vi "Teleop.vi"(10 "Match Info":T1={"Autonomous Elapsed Seconds"=0.0, "TeleOp Elapsed Seconds"=0.0, "Disabled Elapsed Seconds"=0.0, "Visited Autonomous"=FALSE, "Visited TeleOp"=FALSE, "Visited Disabled"=FALSE, "Autonomous Settings"={"Autonomous Style"=enum."Independent", "VI Refnum"=refnum}}, 11 "Call Context":T2) -> ()   [LabVIEW 2014]
doc: "This VI is called for each TeleOp packet received from the DS where the robot is not disabled. It is often used to read from the joysticks and update I/O or to update setpoints for timed control loops. It should complete and return within 20 milliseconds or it may miss DS packets."
uses:
  <vilib>/Rock Robotics/WPI/DriverStation/WPI_DriverStationDerivedRobotMode.ctl
  <vilib>/Rock Robotics/WPI/DriverStation/WPI_DriverStationMatch Info.ctl
  Robot Global Data.vi
  <vilib>/Rock Robotics/WPI/RobotDrive/WPI_RobotDriveMecanumDrive_Cartesian.vi
  <vilib>/Rock Robotics/WPI/Solenoid/Deprecated/WPI_SolenoidSetBool.vi
  <vilib>/Rock Robotics/Network Tables/SD Write Numeric Array.vi
  <vilib>/addons/control/pid/NI_PID_pid.lvlib
  <vilib>/addons/control/pid/pid.llb/PID (DBL).vi
  PID Target Angle.vi
  <vilib>/Rock Robotics/Network Tables/SD Read Boolean.vi
  <vilib>/Rock Robotics/Network Tables/SD Read Number.vi
  <vilib>/Rock Robotics/Network Tables/SD Write Number.vi
panel:
  out "PID Raw Angle":dbl
  out "PID Target":dbl
  out "Joystick Z'":dbl
  out "Joystick Y'":dbl
  out "Joystick X'":dbl
  in  "Lift Encoder Target":dbl
  out "In-Range":bool
  out "Lift Stopped":bool
  out "Lift Direction":bool
  out "Lift Encoder Distance":dbl
  out "Lift Encoder Rate":dbl
  out "Bottom Limit":bool
  out "Top Limit":bool
  out "Wheel Stopped":bool
  out "Wheel Direction":bool
  out "Wheel Encoder Distance":dbl
  out "Wheel Encoder Rate":dbl
  out "Lift Motor Speed":dbl
  out "Angle":dbl(knob) scale=0.0..360.0
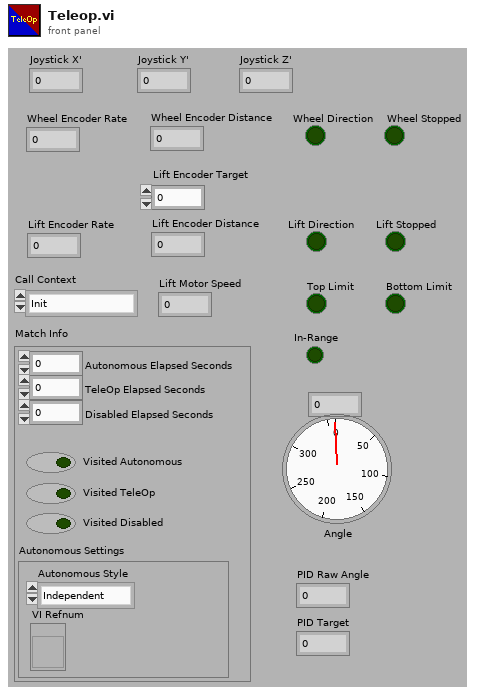
[diagram p1: front panel]
types:
  T1 = typedef "WPI_DriverStationMatch Info.ctl" = cluster{"Autonomous Elapsed Seconds":dbl, "TeleOp Elapsed Seconds":dbl, "Disabled Elapsed Seconds":dbl, "Visited Autonomous":bool, "Visited TeleOp":bool, "Visited Disabled":bool, "Autonomous Settings":cluster{"Autonomous Style":enum16{"Iterative", "Independent"}, "VI Refnum":refnum<vi>}}
  T2 = typedef "WPI_DriverStationDerivedRobotMode.ctl" = enum16{"Init", "Execute", "Stop"}
  T3 = typedef "WPI_GyroDevRef.ctl" = cluster{"DevStatus":errorcluster, "Analog Module":T4, "Analog Channel":T5, "Offset":dbl, "Gain (VoltsPerDegree/Second)":dbl}
  T4 = typedef "FPGA_TypedefAnalogModule.ctl" = enum16{"Controller 1"}
  T5 = typedef "FPGA_AIChannel.ctl" = enum8{"AI 0", "AI 1", "AI 2", "AI 3", "AI MXP 0", "AI MXP 1", "AI MXP 2", "AI MXP 3", "Invalid"}
  T6 = typedef "WPI_JoystickDevRef.ctl" = cluster{"Device":T7}
  T7 = typedef "WPI_JoystickDeviceEnum.ctl" = enum16{"USB 0", "USB 1", "USB 2", "USB 3", "USB 4", "USB 5"}
  T8 = typedef "WPI_SolenoidDevRef.ctl" = cluster{"DevStatus":errorcluster, "Pneumatics Control Module":u8, "Forward Solenoid Channel":T9, "Reverse Solenoid Channel":T9}
  T9 = typedef "WPI_SolenoidChannel.ctl" = enum8{"Solenoid 0", "Solenoid 1", "Solenoid 2", "Solenoid 3", "Solenoid 4", "Solenoid 5", "Solenoid 6", "Solenoid 7", "Invalid"}
  T10 = cluster{"Buttons[0]":bool, "Buttons[1]":bool, "Buttons[2]":bool, "Buttons[3]":bool, "Buttons[4]":bool, "Buttons[5]":bool, "Buttons[6]":bool, "Buttons[7]":bool, "Buttons[8]":bool}
  T11 = typedef "WPI_EncoderDevRef.ctl" = cluster{"DevStatus":errorcluster, "EncoderIndex":T12, "CounterIndex":T13, "DistancePerCount":dbl, "Decoding Type":T14}
  T12 = typedef "FPGA_EncoderIdx.ctl" = enum8{"Enc 0", "Enc 1", "Enc 2", "Enc 3", "Enc 4", "Enc 5", "Enc 6", "Enc 7", "Invalid"}
  T13 = typedef "FPGA_CounterCtrSystemIndex.ctl" = enum8{"Ctr 0", "Ctr 1", "Ctr 2", "Ctr 3", "Ctr 4", "Ctr 5", "Ctr 6", "Ctr 7", "Invalid"}
  T14 = typedef "WPI_EncoderType.ctl" = enum16{"1x", "2x", "4x"}
  T15 = cluster{"proportional gain (Kc)":dbl, "integral time (Ti, min)":dbl, "derivative time (Td, min)":dbl}
  T16 = typedef "WPI_RobotDriveDevRef.ctl" = cluster{"DevStatus":errorcluster, "Motors[]":T17[], "Square Inputs":bool, "Max Output":dbl}
  T17 = typedef "WPI_MotorControlDeviceRef.ctl" = cluster{"DeviceStatus":errorcluster, "Type":T18, "PWM":cluster{"Controller":T19, "PWM Channel":T20, "DeadBand":T21}, "CAN":cluster{"Device Number":u8, "Control Mode":T22, "Semaphore":T23, "Max Vout":dbl, "TalonSRX Control Mode":T24}, "Invert":bool, "TransformRef":T25, "InvTransformRef":T25}
  T18 = typedef "WPI_MotorControlType.ctl" = enum16{"PWM", "CAN", "CANTalonSRX"}
  T19 = typedef "FPGA_TypedefDigitalModule.ctl" = enum16{"Controller 1"}
  T20 = typedef "FPGA_DIOPWMChannel.ctl" = enum8{"PWM 0", "PWM 1", "PWM 2", "PWM 3", "PWM 4", "PWM 5", "PWM 6", "PWM 7", "PWM 8", "PWM 9", "PWM MXP 0", "PWM MXP 1", "PWM MXP 2", "PWM MXP 3", "PWM MXP 4", "PWM MXP 5", "PWM MXP 6", "PWM MXP 7", "PWM MXP 8", "PWM MXP 9", "Invalid"}
  T21 = typedef "WPI_PWMDeadband.ctl" = cluster{"Name":string, "maxPositivePwm":i32, "minPositivePwm":i32, "centerPwm":i32, "maxNegativePwm":i32, "minNegativePwm":i32, "angularRange":u16}
  T22 = typedef "WPI_CANJaguar_ControlMode.ctl" = enum8{"Percent VBus", "Current", "Speed", "Position", "Voltage"}
  T23 = typedef "Semaphore RefNum" = refnum<k1>
  T24 = typedef "WPI_CANTalonSRX_APIControlMode.ctl" = enum8{"Percent VBus", "Speed", "Position", "Slave", "Unchanged / Invalid"}
  T25 = typedef "WPI_PWMTransform_ConPane.ctl" = refnum<vi>
  T26 = typedef "WPI_SwitchDevRef.ctl" = cluster{"DevStatus":errorcluster, "DIO Channel":T27, "Controller":T19, "CntIndex":T13, "Normally Closed":bool}
  T27 = typedef "FPGA_DIOChannel.ctl" = enum8{"DIO 0", "DIO 1", "DIO 2", "DIO 3", "DIO 4", "DIO 5", "DIO 6", "DIO 7", "DIO 8", "DIO 9", "DIO MXP 0", "DIO MXP 1", "DIO MXP 2", "DIO MXP 3", "DIO MXP 4", "DIO MXP 5", "DIO MXP 6", "DIO MXP 7", "DIO MXP 8", "DIO MXP 9", "DIO MXP 10", "DIO MXP 11", "DIO MXP 12", "DIO MXP 13", "DIO MXP 14", "DIO MXP 15", "Invalid"}
  T28 = cluster{"X":dbl, "Y":dbl, "Angle":dbl, "Magnitude":dbl}
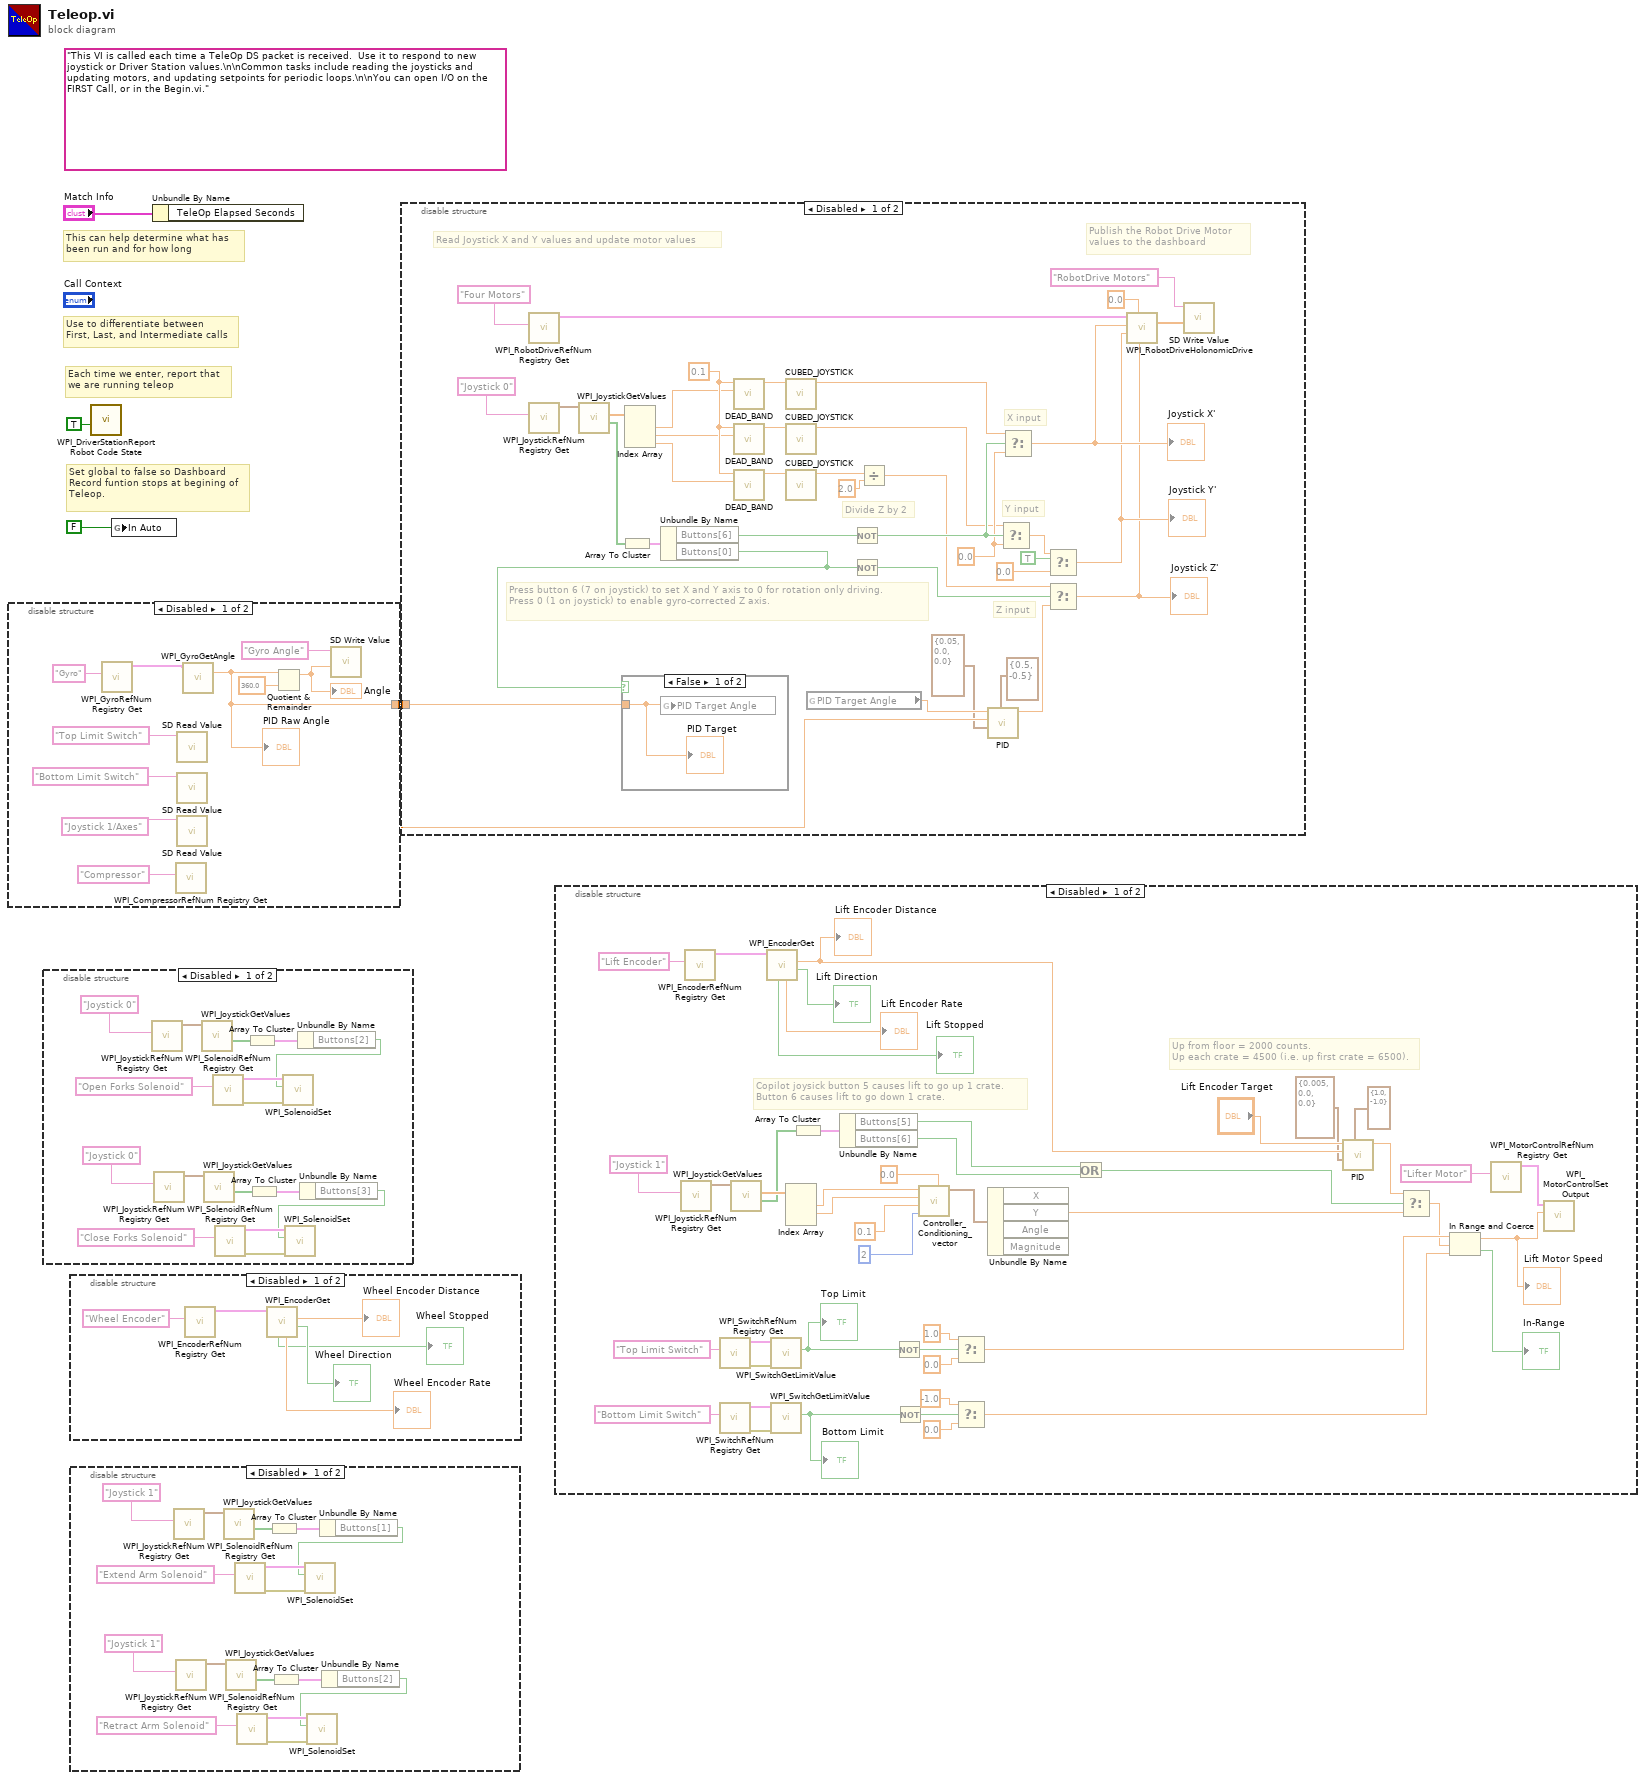
[diagram p0: block diagram]
diagram:
  (unwired) "This VI is called each time a TeleOp DS packet is received.  Use it to respond to new joystick or Driver Station values.\n\nCommon tasks include reading the joysticks and updating motors, and updating setpoints for periodic loops.\n\nYou can open I/O on the FIRST Call, or in the Begin.vi."
  # "Set global to false so Dashboard Record funtion stops at begining of Teleop."
  # "Each time we enter, report that\nwe are running teleop"
  # "Use to differentiate between\nFirst, Last, and Intermediate calls"
  # "This can help determine what has\nbeen run and for how long"
  n1 = disable-structure shown="Disabled" {
    disable-tunnel: [w6 _] -> w2
    frame Disabled {
      n2 = call <vilib>:"WPI_GyroRefNum Registry Get.vi"("refnum name"="Gyro") -> ("GyroDevRef"=w8:T3)  [unwired: 9 in, 1 out]
      n3 = call <vilib>:"WPI_CompressorRefNum Registry Get.vi"("refnum name"="Compressor") -> ()  [unwired: 9 in, 2 out]
      n4 = call-poly <vilib>:"SD Read Value.vi"("Name"="Top Limit Switch" ("refnum name")) -> ()  [unwired: 8 in, 3 out]
      n5 = call-poly <vilib>:"SD Read Value.vi"("Name"="Bottom Limit Switch" ("refnum name")) -> ()  [unwired: 8 in, 3 out]
      n6 = call-poly <vilib>:"SD Read Value.vi"("Name"="Joystick 1/Axes" ("refnum name")) -> ()  [unwired: 8 in, 3 out]
      n7 = call <vilib>:"WPI_GyroGetAngle.vi"("GyroDevRef"=w8) -> ("Angle"=w6:dbl)  [unwired: 7 in, 3 out]
      "PID Raw Angle" <- w6
      n8 = Quotient & Remainder(x=w6, y=360.0) -> (x-y*floor(x/y)=w7:dbl)  [unwired: 1 out]
      "Angle" <- w7
      n9 = call-poly <vilib>:"SD Write Value.vi"("Numeric"=w7, "Name"="Gyro Angle") -> ()  [unwired: 8 in, 2 out]
    }
    frame Enabled {
    }
  }
  n10 = disable-structure shown="Disabled" {
    frame Disabled {
      n11 = call <vilib>:"WPI_JoystickRefNum Registry Get.vi"("refnum name"="Joystick 0") -> ("JoystickDevRef"=w29:T6)  [unwired: 1 in, 9 out]
      n12 = call <vilib>:"WPI_JoystickRefNum Registry Get.vi"("refnum name"="Joystick 0") -> ("JoystickDevRef"=w22:T6)  [unwired: 1 in, 9 out]
      n13 = call <vilib>:"WPI_JoystickGetValues.vi"("JoystickDevRef"=w29) -> ("Buttons"=w25:bool[])  [unwired: 6 in, 4 out]
      n14 = call <vilib>:"WPI_JoystickGetValues.vi"("JoystickDevRef"=w22) -> ("Buttons"=w18:bool[])  [unwired: 6 in, 4 out]
      n15 = call <vilib>:"WPI_SolenoidRefNum Registry Get.vi"("refnum name"="Open Forks Solenoid") -> ("error out"=w28:errorcluster, "SolenoidDevRef"=w27:T8)  [unwired: 9 in]
      n16 = call <vilib>:"WPI_SolenoidRefNum Registry Get.vi"("refnum name"="Close Forks Solenoid") -> ("error out"=w21:errorcluster, "SolenoidDevRef"=w20:T8)  [unwired: 9 in]
      n17 = Array To Cluster(array=w25) -> (cluster=w24:T10)
      n18 = Array To Cluster(array=w18) -> (cluster=w17:T10)
      n19 = Unbundle By Name(w24) -> ("Buttons[2]"=w15:bool)
      n20 = call-poly <vilib>:"WPI_SolenoidSet.vi"("error in (no error)"=w28, "Value"=w15, "SolenoidDevRef"=w27) -> ()  [unwired: 7 in, 2 out]
      n21 = Unbundle By Name(w17) -> ("Buttons[3]"=w16:bool)
      n22 = call-poly <vilib>:"WPI_SolenoidSet.vi"("error in (no error)"=w21, "Value"=w16, "SolenoidDevRef"=w20) -> ()  [unwired: 7 in, 2 out]
    }
    frame Enabled {
    }
  }
  n23 = disable-structure shown="Disabled" {
    frame Disabled {
      n24 = call <vilib>:"WPI_EncoderRefNum Registry Get.vi"("refnum name"="Wheel Encoder") -> ("EncoderDevRef"=w35:T11)  [unwired: 9 in, 1 out]
      n25 = call <vilib>:"WPI_EncoderGet.vi"("EncoderDevRef"=w35) -> ("Direction"=→"Wheel Direction":bool, "Distance"=→"Wheel Encoder Distance":dbl, "Rate"=→"Wheel Encoder Rate":dbl, "Stopped"=→"Wheel Stopped":bool)  [unwired: 5 in, 2 out]
    }
    frame Enabled {
    }
  }
  n26 = disable-structure shown="Disabled" {
    frame Disabled {
      n27 = call <vilib>:"WPI_JoystickRefNum Registry Get.vi"("refnum name"="Joystick 1") -> ("JoystickDevRef"=w51:T6)  [unwired: 1 in, 9 out]
      n28 = call <vilib>:"WPI_JoystickRefNum Registry Get.vi"("refnum name"="Joystick 1") -> ("JoystickDevRef"=w44:T6)  [unwired: 1 in, 9 out]
      n29 = call <vilib>:"WPI_JoystickGetValues.vi"("JoystickDevRef"=w51) -> ("Buttons"=w47:bool[])  [unwired: 6 in, 4 out]
      n30 = call <vilib>:"WPI_JoystickGetValues.vi"("JoystickDevRef"=w44) -> ("Buttons"=w40:bool[])  [unwired: 6 in, 4 out]
      n31 = call <vilib>:"WPI_SolenoidRefNum Registry Get.vi"("refnum name"="Extend Arm Solenoid") -> ("error out"=w50:errorcluster, "SolenoidDevRef"=w49:T8)  [unwired: 9 in]
      n32 = call <vilib>:"WPI_SolenoidRefNum Registry Get.vi"("refnum name"="Retract Arm Solenoid") -> ("error out"=w43:errorcluster, "SolenoidDevRef"=w42:T8)  [unwired: 9 in]
      n33 = Array To Cluster(array=w47) -> (cluster=w46:T10)
      n34 = Array To Cluster(array=w40) -> (cluster=w39:T10)
      n35 = Unbundle By Name(w46) -> ("Buttons[1]"=w37:bool)
      n36 = call-poly <vilib>:"WPI_SolenoidSet.vi"("error in (no error)"=w50, "Value"=w37, "SolenoidDevRef"=w49) -> ()  [unwired: 7 in, 2 out]
      n37 = Unbundle By Name(w39) -> ("Buttons[2]"=w38:bool)
      n38 = call-poly <vilib>:"WPI_SolenoidSet.vi"("error in (no error)"=w43, "Value"=w38, "SolenoidDevRef"=w42) -> ()  [unwired: 7 in, 2 out]
    }
    frame Enabled {
    }
  }
  n39 = call <vilib>:"WPI_DriverStationReport Robot Code State.vi"("TeleOp"=TRUE ("Autonomous")) -> ()  [unwired: 10 in, 1 out]
  n40 = global write "Robot Global Data.vi" "In Auto"(FALSE) -> ()
  n41 = Unbundle By Name("Match Info") -> ()  [unwired: 1 out]
  n42 = disable-structure shown="Disabled" {
    disable-tunnel: w2 -> [w55 _]
    frame Disabled {
      w73 = 0.1 ("deadband input")
      w80 = 0.0
      # "Divide Z by 2"
      # "Z input"
      # "Y input"
      # "X input"
      # "Press button 6 (7 on joystick) to set X and Y axis to 0 for rotation only driving.\nPress 0 (1 on joystick) to enable gyro-corrected Z axis."
      # "Publish the Robot Drive Motor\nvalues to the dashboard"
      # "Read Joystick X and Y values and update motor values"
      n43 = call <vilib>:"WPI_RobotDriveRefNum Registry Get.vi"("refnum name"="Four Motors") -> ("RobotDriveDevRef"=w89:T16)  [unwired: 1 in, 9 out]
      n44 = call <vilib>:"WPI_JoystickRefNum Registry Get.vi"("refnum name"="Joystick 0") -> ("JoystickDevRef"=w87:T6)  [unwired: 1 in, 9 out]
      n45 = call <vilib>:"WPI_JoystickGetValues.vi"("JoystickDevRef"=w87) -> ("Buttons"=w67:bool[], "Axes"=w84:dbl[])  [unwired: 6 in, 3 out]
      n46 = Array To Cluster(array=w67) -> (cluster=w83:T10)
      n47 = Index Array(array=w84) -> (element #1=w71:dbl, element #2=w70:dbl, element #3=w69:dbl)  [unwired: 3 in]
      n48 = Unbundle By Name(w83) -> ("Buttons[6]"=w82:bool, "Buttons[0]"=w57:bool)
      n49 = case shown="False" w57 {
        tunnel: w55 -> [w91 _]
        frame False {
          n50 = global write "PID Target Angle.vi" "PID Target Angle"(w91) -> ()
          "PID Target" <- w91
        }
        frame True {
        }
      }
      n51 = call "DEAD_BAND.vi"("axis input"=w71, "deadband input"=w73) -> ("axis output"=w76:dbl)  [unwired: 9 in]
      n52 = call "DEAD_BAND.vi"("axis input"=w70, "deadband input"=w73) -> ("axis output"=w75:dbl)  [unwired: 9 in]
      n53 = call "DEAD_BAND.vi"("axis input"=w69, "deadband input"=w73) -> ("axis output"=w74:dbl)  [unwired: 9 in]
      n54 = call "CUBED_JOYSTICK.vi"("axis input"=w76) -> ("axis output"=w72:dbl)  [unwired: 10 in]
      n55 = call "CUBED_JOYSTICK.vi"("axis input"=w75) -> ("axis output"=w68:dbl)  [unwired: 10 in]
      n56 = call "CUBED_JOYSTICK.vi"("axis input"=w74) -> ("axis output"=w60:dbl)  [unwired: 10 in]
      n57 = global read "PID Target Angle.vi" "PID Target Angle"() -> (w56:dbl)
      n58 = Not(x=w82) -> (.not. x?=w81:bool)
      n59 = Not(x=w57) -> (.not. x?=w78:bool)
      n60 = Divide(x=w60, y=2.0) -> (x/y=w59:dbl)
      n61 = call-poly <vilib>:"PID.vi"("output range"=cluster{"output high":dbl, "output low":dbl} {"output high"=0.5, "output low"=-0.5}, "PID gains"=T15 {"proportional gain (Kc)"=0.05, "integral time (Ti, min)"=0.0, "derivative time (Td, min)"=0.0}, "process variable"=w55, "setpoint"=w56) -> ("output"=w62:dbl)  [unwired: 6 in, 1 out]
      n62 = Select(t=w68, s=w81, f=w80) -> (s? t:f=w77:dbl)
      n63 = Select(t=w72, s=w81, f=w80) -> (s? t:f=w66:dbl)
      "Joystick X'" <- w66
      n64 = Select(t=w77, s=TRUE, f=0.0) -> (s? t:f=w65:dbl)
      "Joystick Y'" <- w65
      n65 = Select(t=w59, s=w78, f=w62) -> (s? t:f=w58:dbl)
      "Joystick Z'" <- w58
      n66 = call-poly <vilib>:"WPI_RobotDriveHolonomicDrive.vi"("Rotation"=w58, "Gyro Angle"=0.0, "Y"=w65, "X"=w66, "RobotDriveDevRef"=w89) -> ("Motor Values"=w85:dbl[])  [unwired: 4 in, 2 out]
      n67 = call-poly <vilib>:"SD Write Value.vi"("Numeric Array"=w85, "Name"="RobotDrive Motors") -> ()  [unwired: 8 in, 2 out]
    }
    frame Enabled {
    }
  }
  n68 = disable-structure shown="Disabled" {
    frame Disabled {
      # "Up from floor = 2000 counts.\nUp each crate = 4500 (i.e. up first crate = 6500)."
      # "Copilot joysick button 5 causes lift to go up 1 crate.\nButton 6 causes lift to go down 1 crate."
      n69 = call <vilib>:"WPI_JoystickRefNum Registry Get.vi"("refnum name"="Joystick 1") -> ("JoystickDevRef"=w136:T6)  [unwired: 1 in, 9 out]
      n70 = call <vilib>:"WPI_EncoderRefNum Registry Get.vi"("refnum name"="Lift Encoder") -> ("EncoderDevRef"=w113:T11)  [unwired: 9 in, 1 out]
      n71 = call <vilib>:"WPI_SwitchRefNum Registry Get.vi"("refnum name"="Top Limit Switch") -> ("error out"=w124:errorcluster, "SwitchDevRef"=w125:T26)  [unwired: 9 in]
      n72 = call <vilib>:"WPI_SwitchRefNum Registry Get.vi"("refnum name"="Bottom Limit Switch") -> ("error out"=w121:errorcluster, "SwitchDevRef"=w122:T26)  [unwired: 9 in]
      n73 = call <vilib>:"WPI_JoystickGetValues.vi"("JoystickDevRef"=w136) -> ("Buttons"=w103:bool[], "Axes"=w135:dbl[])  [unwired: 6 in, 3 out]
      n74 = call <vilib>:"WPI_EncoderGet.vi"("EncoderDevRef"=w113) -> ("Direction"=→"Lift Direction":bool, "Distance"=w94:dbl, "Rate"=→"Lift Encoder Rate":dbl, "Stopped"=→"Lift Stopped":bool)  [unwired: 5 in, 2 out]
      "Lift Encoder Distance" <- w94
      n75 = call <vilib>:"WPI_SwitchGetLimitValue.vi"("error in (no error)"=w124, "SwitchDevRef"=w125) -> ("Switch Pressed"=w107:bool)  [unwired: 7 in, 2 out]
      "Top Limit" <- w107
      n76 = call <vilib>:"WPI_SwitchGetLimitValue.vi"("error in (no error)"=w121, "SwitchDevRef"=w122) -> ("Switch Pressed"=w105:bool)  [unwired: 7 in, 2 out]
      "Bottom Limit" <- w105
      n77 = Index Array(array=w135) -> (element #1=w134:dbl, element #2=w133:dbl)  [unwired: 3 in, 1 out]
      n78 = Array To Cluster(array=w103) -> (cluster=w102:T10)
      n79 = Unbundle By Name(w102) -> ("Buttons[5]"=w97:bool, "Buttons[6]"=w98:bool)
      n80 = Not(x=w107) -> (.not. x?=w106:bool)
      n81 = Not(x=w105) -> (.not. x?=w104:bool)
      n82 = call "Controller_Conditioning_vector.vi"("Min Output(0 to 1)"=0.0, "Enum"=2, "Dead Zone(0 to 1)"=0.1, "Y(-1 to 1)"=w133, "X(-1 to 1)"=w134) -> ("output cluster"=w132:T28)  [unwired: 6 in]
      n83 = Select(t=1.0, s=w106, f=0.0 ("t")) -> (s? t:f=w116:dbl)
      n84 = Select(t=-1.0, s=w104, f=0.0 ("t")) -> (s? t:f=w115:dbl)
      n85 = Unbundle By Name(w132) -> ("Y"=w100:dbl)  [unwired: 3 out]
      n86 = Or(x=w97, y=w98) -> (x .or. y?=w99:bool)
      n87 = call-poly <vilib>:"PID.vi"("output range"=cluster{"output high":dbl, "output low":dbl} {"output high"=1.0, "output low"=-1.0}, "PID gains"=T15 {"proportional gain (Kc)"=0.005, "integral time (Ti, min)"=0.0, "derivative time (Td, min)"=0.0}, "process variable"=w94, "setpoint"="Lift Encoder Target") -> ("output"=w96:dbl)  [unwired: 6 in, 1 out]
      n88 = Select(t=w96, s=w99, f=w100) -> (s? t:f=w101:dbl)
      n89 = In Range and Coerce(upper limit=w116, x=w101, lower limit=w115) -> (coerced(x)=w108:dbl, In Range?=→"In-Range":bool)
      "Lift Motor Speed" <- w108
      n90 = call <vilib>:"WPI_MotorControlRefNum Registry Get.vi"("refnum name"="Lifter Motor") -> ("MotorControlDevRef"=w128:T17)  [unwired: 9 in, 1 out]
      n91 = call <vilib>:"WPI_MotorControlSetOutput.vi"("Output"=w108, "MotorControlDevRef"=w128) -> ()  [unwired: 7 in, 3 out]
    }
    frame Enabled {
    }
  }
